vi "Read Headers.vi"(7 "Linked List ID":string, 8 "error in (no error)":errorcluster, 11 "Linked List Ref":refnum<data-value>) -> (0 "error out":errorcluster, 1 "Header Values":string[](array[string]), 2 "Header Names":string[](array[string]), 3 "Linked List Ref out":refnum<data-value>, 4 "found":bool)   [LabVIEW 2020, in "Linked Lists.lvlib" / "Linked List Ref.lvclass"]
uses:
  <vilib>/gpm_packages/@cs/linked-list/Source/Linked List/Linked List Ref/Linked List Ref.lvclass
  <vilib>/gpm_packages/@cs/linked-list/Source/Linked List/ILinkedList/ILinked List.lvclass
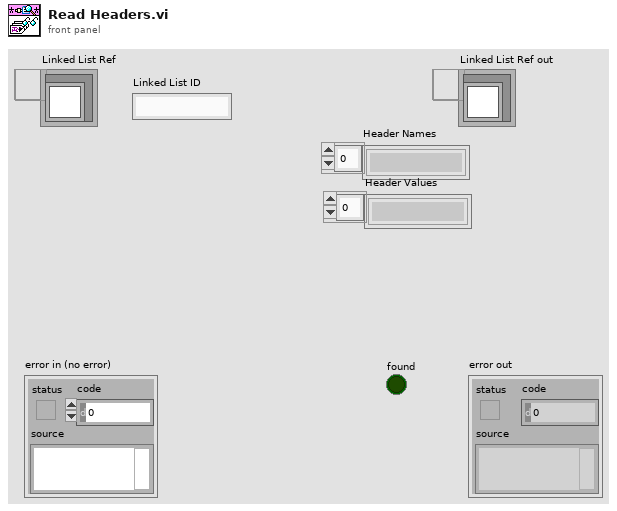
[diagram p1: front panel]
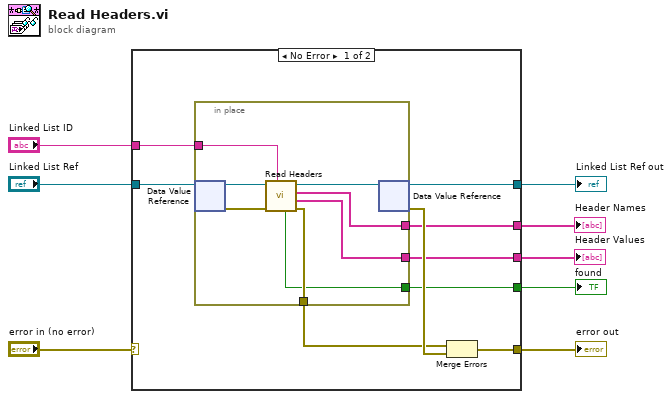
[diagram p0: block diagram]
diagram:
  n1 = case shown="No Error" "error in (no error)" {
    selector: "error in (no error)" -> [_ w27]
    tunnel: "Linked List Ref" -> [w17 w26]
    tunnel: "Linked List ID" -> [w16 _]
    tunnel: [w14 w27] -> w5
    tunnel: [w15 w26] -> w4
    tunnel: [w11 _] -> w3
    tunnel: [w10 _] -> w2
    tunnel: [w9 _] -> w1
    frame No Error {
      n2 = in-place {
        in-place-border: w16 -> [w23]
        in-place-border: [w21] -> w12
        in-place-border: [w20] -> w11
        in-place-border: [w19] -> w10
        in-place-border: [w18] -> w9
        n3 = in-place-dvr #1(w17) -> (w25:refnum<class "ILinked List.lvclass">, w22:errorcluster)
        n4 = call-dynamic "Read Headers.vi"("Linked List ID"=w23, "error in (no error)"=w22, "ILinked List in"=w25) -> ("error out"=w21:errorcluster, "Header Values"=w18:string[], "Header Names"=w19:string[], "ILinked List out"=w24:refnum<class "ILinked List.lvclass">, "found"=w20:bool)  [unwired: 4 in]
        n5 = in-place-dvr #1(w24) -> (w15:refnum<data-value>, w13:errorcluster)
      }
      n6 = Merge Errors(w12, w13) -> (w14:errorcluster)
    }
    frame Error {
    }
  }
  "error out" <- w5
  "Linked List Ref out" <- w4
  "found" <- w3
  "Header Names" <- w2
  "Header Values" <- w1
